vi "robotOrientedToPoint.vi"(8 "error in (no error)":errorcluster, 9 "Target":dbl[](array[numeric]), 10 "Robot":refnum<class "Robot.lvclass">, 11 "Utilities in":refnum<class "Utilities.lvclass">) -> (0 "error out":errorcluster, 2 "Orientation":dbl, 3 "Utilities out":refnum<class "Utilities.lvclass">)   [LabVIEW 2023, in "Utilities.lvclass"]
uses:
  Utilities.lvclass
  Robot_class/Robot.lvclass
  C:/Users/ebert/Desktop/roboime/SSL_AI/Object_class/Object.lvclass
  Object_class/Object.lvclass/Object.ctl
  Object_class/Read x.vi
  Object_class/Read y.vi
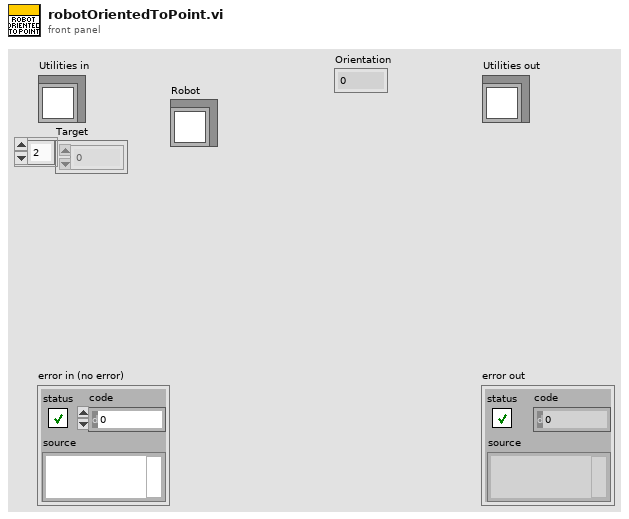
[diagram p1: front panel]
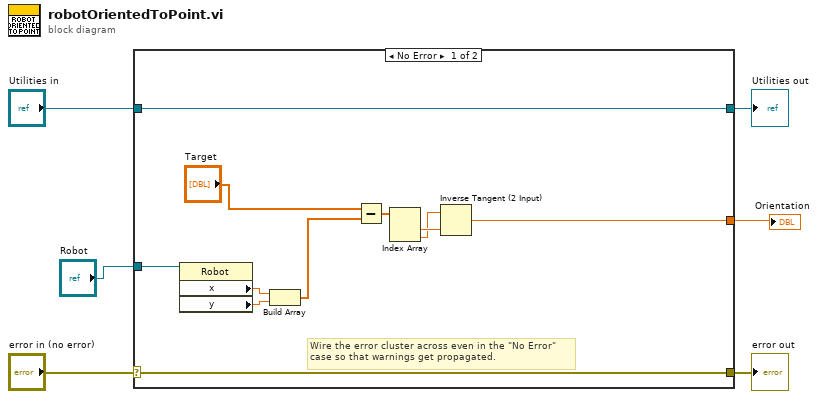
[diagram p0: block diagram]
diagram:
  n1 = case shown="No Error" "error in (no error)" {
    selector: "error in (no error)" -> [w16 w19]
    tunnel: [w16 w19] -> w5
    tunnel: [w17 w18] -> w3
    tunnel: "Utilities in" -> [w17 w18]
    tunnel: "Robot" -> [w13 _]
    tunnel: [w7 _] -> w1
    frame No Error {
      # "Wire the error cluster across even in the \"No Error\"\ncase so that warnings get propagated."
      n2 = property class="Robot"(reference=w13) -> ("x"=w15:dbl, "y"=w14:dbl)  [unwired: 1 in, 2 out]
      n3 = Build Array(w15, w14) -> (w9:dbl[])
      n4 = Subtract(x="Target", y=w9) -> (x-y=w12:dbl[])
      n5 = Index Array(array=w12) -> (element #1=w11:dbl, element #2=w10:dbl)  [unwired: 2 in]
      n6 = Inverse Tangent (2 Input)(1:w11, 2:w10) -> (0:w7:dbl)
    }
    frame Error {
    }
  }
  "error out" <- w5
  "Utilities out" <- w3
  "Orientation" <- w1
